vi "Timed and Median Output Analog Input.vi"(8 "error in (no error)":errorcluster, 10 "Time to collect [ms]":i32=100, 11 "Channel":i32) -> (0 "error out":errorcluster, 3 "Median of timed measurement [v]":dbl format="%0.2f")   [LabVIEW 2016]
uses:
  <vilib>/Analysis/NI_AALBase.lvlib
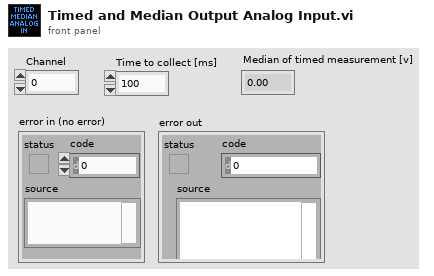
[diagram p1: front panel]
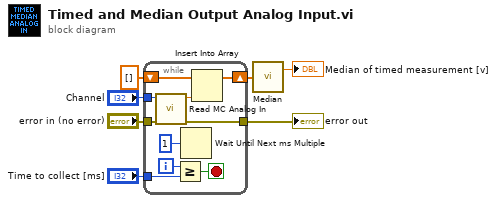
[diagram p0: block diagram]
diagram:
  n1 = while {
    shift-right: [w10] -> w5
    shift-left: dbl[] [] -> [w16]
    tunnel: "Channel" -> [w15]
    tunnel: "Time to collect [ms]" -> [w11]
    tunnel: "error in (no error)" -> [w9]
    tunnel: [w8] -> w1
    i -> [w13]
    stop <- w12 stop-if-true
    n2 = call "Read MC Analog In.vi"("error in (no error)"=w9, "channel"=w15) -> ("error out"=w8:errorcluster, "Voltage Input"=w17:dbl)  [unwired: 8 in]
    n3 = Greater Or Equal?(x=w13, y=w11) -> (x >= y?=w12:bool)
    n4 = Wait Until Next ms Multiple(millisecond multiple=u32 1) -> ()  [unwired: 1 out]
    n5 = Insert Into Array(array=w16, new element=w17) -> (w10:dbl[])  [unwired: 1 in]
  }
  "error out" <- w1
  n6 = call <vilib>:"Median.vi"("X"=w5) -> ("median"=→"Median of timed measurement [v]":dbl)  [unwired: 1 out]
